vi "DMM.vi"() -> ()   [LabVIEW 2017]
panel:
  in  "Slide":u8(slide)=255 scale=0.0..255.0
  in  "Stop Button":bool
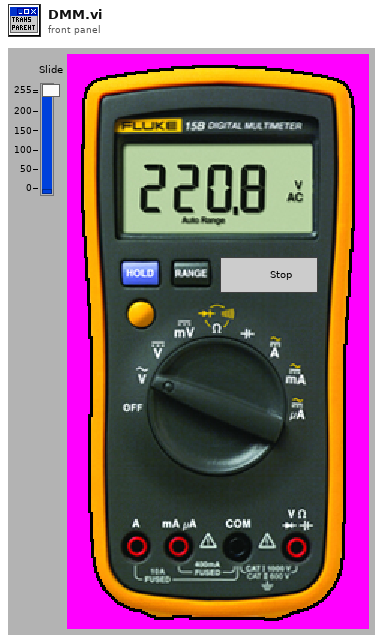
[diagram p1: front panel]
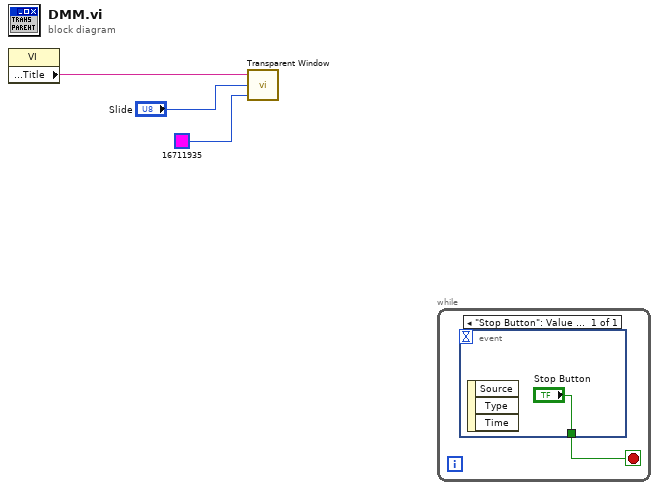
[diagram p0: block diagram]
diagram:
  n1 = property class="VI"() -> ("Front Panel.Title"=w1:string)  [unwired: 2 in, 2 out]
  n2 = call "Transparent Window.vi"("crkey"=u32 16711935 ("Color Box"), "Slide"="Slide", "window name (\"\")"=w1) -> ()  [unwired: 1 in]
  n3 = while {
    stop <- w4 stop-if-true
    n4 = event shown="[0] \"Stop Button\": Value Change" {
      selector: _ -> [_]
      dyn-events: _ -> [_]
      timeout: _ -> [_]
      tunnel: ["Stop Button"] -> w4
      event "Stop Button": Value Change {
        n5 = event-data() -> ()  [unwired: 1 in, 3 out]
      }
    }
  }
